vi "Sample_Finite.vi"() -> ()   [LabVIEW 2013]
doc: "This samples demonstrates how to sample a finite waveform."
uses:
  <userlib>/ArtScope/Trigger/ArtScope_ConfigureTriggerSoftWare.vi
  <userlib>/ArtScope/Fetch/ArtScope_FetchVoltage.vi
  <userlib>/ArtScope/_SubVI/ArtScope_ArrayByChannel_DBL.vi
panel:
  in  "reference position":dbl
  in  "range(Vpp)":i32(ring) items=["20V", "10V", "2V", "40V", "16V", "8V", "4V", "1.6V", "800m", "400m", "160m", "80m", "40m"]
  in  "offset(mV)":i32
  in  "num samples":i32=1000
  in  "Stop":bool
  out "waveform":dbl[][](graph)
  out "error out":errorcluster={"status"=FALSE, "code"=0, "source"="\n"}
  in  "timeout(s)":dbl=10.0
  in  "min record length":i32=6000
  in  "min sample rate":dbl=800000.0
  in  "coupling":i32(ring) items=["DC", "AC"]
  in  "channel name":string="0"
  in  "resource name":string="Dev1"
  # "Vertical"
  # "Horizontal"
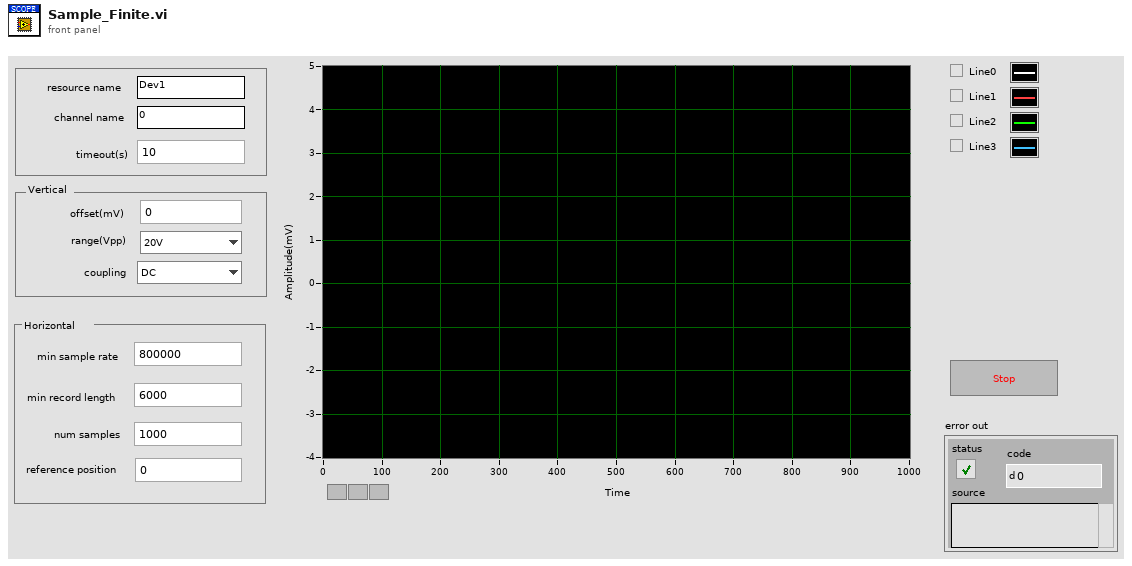
[diagram p1: front panel]
types:
  T1 = cluster{"fLSB":cluster{dbl, dbl, dbl, dbl, dbl, dbl, dbl, dbl}, "RangeValue":cluster{dbl, dbl, dbl, dbl, dbl, dbl, dbl, dbl}, "wMaxLSB":u32, "TriggerMode":i32, "sampLengthPerChan":u32, "pAvailSampsPoints":u32, "channelCount":i32}
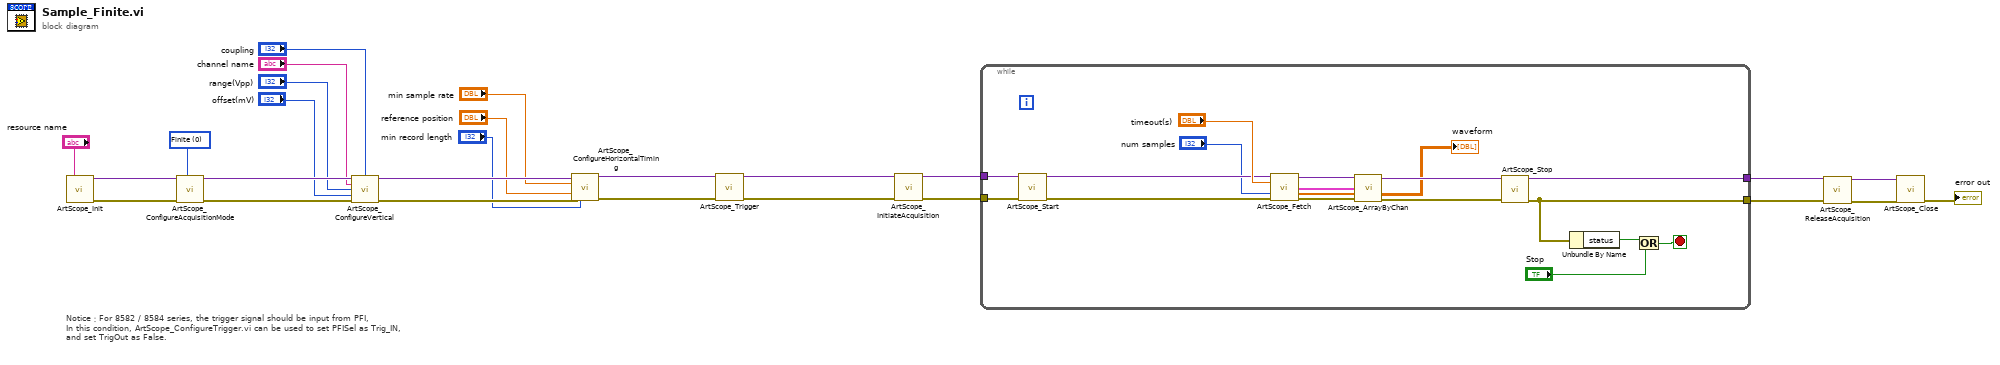
[diagram p0: block diagram]
diagram:
  w18 = 0 items=["Finite", "Continuous"] ("AcuqMode")
  # "Notice：For 8582 / 8584 series, the trigger signal should be input from PFI, \nIn this condition, ArtScope_ConfigureTrigger.vi can be used to set PFISel as Trig_IN,\nand set TrigOut as False."
  n1 = call <userlib>:"ArtScope_Init.vi"("task name"="resource name") -> ("task handle"=w19:variant, "error out"=w20:errorcluster)  [unwired: 13 in]
  n2 = call <userlib>:"ArtScope_ConfigureAcquisitionMode.vi"("task handle"=w19, "acquisition mode"=w18, "error in (no error)"=w20) -> ("task handle"=w17:variant, "error out"=w21:errorcluster)  [unwired: 11 in]
  n3 = call <userlib>:"ArtScope_ConfigureVertical.vi"("task handle"=w17, "coupling"="coupling", "channels"="channel name", "range(Vpp)"="range(Vpp)", "offset"="offset(mV)", "error in (no error)"=w21) -> ("task handle"=w24:variant, "error out"=w23:errorcluster)  [unwired: 8 in]
  n4 = call <userlib>:"ArtScope_ConfigureHorizontalTiming.vi"("task handle"=w24, "min sample rate"="min sample rate", "reference position"="reference position", "error in (no error)"=w23, "min record length"="min record length") -> ("task handle"=w15:variant, "error out"=w16:errorcluster)  [unwired: 9 in]
  n5 = call-poly <userlib>:"ArtScope_Trigger.vi"("task handle"=w15, "error in (no error)"=w16) -> ("task handle"=w7:variant, "error out"=w6:errorcluster)  [unwired: 12 in]
  n6 = call <userlib>:"ArtScope_InitiateAcquisition.vi"("task handle"=w7, "error in (no error)"=w6) -> ("task handle"=w5:variant, "error out"=w4:errorcluster)  [unwired: 12 in]
  n7 = while {
    tunnel: [w40] -> w11
    tunnel: [w39] -> w10
    tunnel: w5 -> [w38]
    tunnel: w4 -> [w43]
    stop <- w41 stop-if-true
    n8 = call <userlib>:"ArtScope_Start.vi"("task handle"=w38, "error in (no error)"=w43) -> ("task handle"=w36:variant, "error out"=w35:errorcluster)  [unwired: 12 in]
    n9 = call-poly <userlib>:"ArtScope_Fetch.vi"("task handle"=w36, "timeout"="timeout(s)", "num samples"="num samples", "error in (no error)"=w35) -> ("task handle"=w30:variant, "wfm info"=w29:T1, "data"=w28:dbl[], "error out"=w33:errorcluster)  [unwired: 8 in]
    n10 = call-poly <userlib>:"ArtScope_ArrayByChan.vi"("task handle"=w30, "wfm info"=w29, "1D data"=w28, "error in (no error)"=w33) -> ("task handle"=w31:variant, "2D data"=→"waveform":dbl[][], "error out"=w32:errorcluster)  [unwired: 9 in]
    n11 = call <userlib>:"ArtScope_Stop.vi"("task handle"=w31, "error in (no error)"=w32) -> ("task handle"=w40:variant, "error out"=w39:errorcluster)  [unwired: 12 in]
    n12 = Unbundle By Name(w39) -> ("status"=w42:bool)
    n13 = Or(x=w42, y="Stop") -> (x .or. y?=w41:bool)
  }
  n14 = call <userlib>:"ArtScope_ReleaseAcquisition.vi"("task handle"=w11, "error in (no error)"=w10) -> ("task handle"=w9:variant, "error out"=w8:errorcluster)  [unwired: 12 in]
  n15 = call <userlib>:"ArtScope_Close.vi"("task handle"=w9, "error in (no error)"=w8) -> ("error out"=→"error out":errorcluster)  [unwired: 13 in]
